vi "Host_UDPGLOBALS.vi"() -> ()   [LabVIEW 2018]
panel:
  out "UDP Sent?":bool
  in  "IP Address":string="192.168.0.1"
  in  "UDP String":string
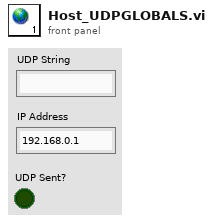
[diagram p1: front panel]
diagram:
